vi "Lab Panel Global 1.vi"() -> ()   [LabVIEW 2013]
panel:
  out "Numeric Indicator":dbl
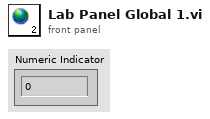
[diagram p1: front panel]
diagram:
